vi "Get_ini_KEY.vi"(8 "error in (no error)":errorcluster caption="错误输入（无错误）", 10 "key":string caption="键", 11 "section":string caption="段") -> (0 "error out":errorcluster, 2 "value":string)   [LabVIEW 2018]
uses:
  Global.vi
  <vilib>/Utility/config.llb/Read Key (String).vi
  <vilib>/Utility/config.llb/NI_LVConfig.lvlib
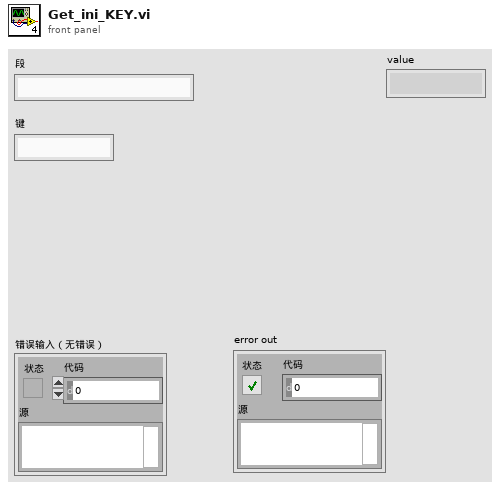
[diagram p1: front panel]
types:
  T1 = typedef "NI_LVConfig.lvlib/Config Data RefNum.ctl" = refnum<k1>
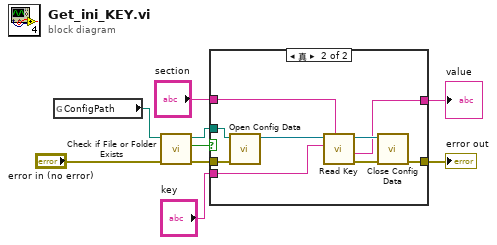
[diagram p0: block diagram]
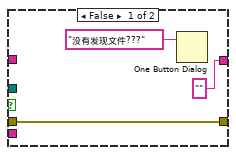
[diagram p2: hidden frame]
diagram:
  n1 = global read "Global.vi" "ConfigPath"() -> (w9:path)
  n2 = call <vilib>:"Check if File or Folder Exists.vi"("error in (no error)"="error in (no error)", "path"=w9) -> ("error out"=w5:errorcluster, "file or folder exists?"=w7:bool, "dup path"=w8:path)  [unwired: 7 in]
  n3 = case shown="真" w7 {
    tunnel: w8 -> [_ w21]
    tunnel: "section" -> [_ w20]
    tunnel: ["" w14] -> w1
    tunnel: w5 -> [w11 w19]
    tunnel: [w11 w16] -> w4
    tunnel: "key" -> [_ w15]
    frame False {
      n4 = One Button Dialog(message="没有发现文件???" ("消息")) -> ()  [unwired: 1 in, 1 out]
    }
    frame True {
      n5 = call <vilib>:"Open Config Data.vi"("error in (no error)"=w19, "configuration file path"=w21) -> ("refnum"=w13:T1)  [unwired: 7 in, 2 out]
      n6 = call-poly <vilib>:"Read Key.vi"("section"=w20, "key"=w15, "refnum"=w13) -> ("error out"=w17:errorcluster, "value"=w14:string, "refnum out"=w18:T1)  [unwired: 5 in, 1 out]
      n7 = call <vilib>:"Close Config Data.vi"("error in (no error)"=w17, "refnum"=w18) -> ("error out"=w16:errorcluster)  [unwired: 8 in, 1 out]
    }
  }
  "error out" <- w4
  "value" <- w1
